vi "O2Scale.vi"() -> ()   [LabVIEW 2018]
uses:
  <vilib>/regexp/Match Regular Expression.xnode
panel:
  out "data out init 4":string="53 Ready for user\r\n"
  out "data out init 3":string="12 Access OK\r\n"
  in  "address 2":string="192.168.1.102"
  out "data out 4":string="00R614~       641.0~\r\n"
  in  "bytes to read 2":i32=100
  out "data out 3":string="00R615~       252.0~\r\n"
  out "East Scale\nWeight [lbs] 2":dbl(knob)=641.0 scale=0.0..800.0
  out "O2 East\nWeight [lbs] 2":dbl(knob)=252.0 scale=0.0..600.0
  out "O2 West\nWeight [lbs]":dbl(knob)=252.0 scale=0.0..600.0
  out "West Scale\nWeight [lbs]":dbl(knob)=641.0 scale=0.0..800.0
  in  "address":string="192.168.1.101"
  out "data out 2":string="00R131~       252.0~\r\n"
  in  "bytes to read":i32=100
  in  "stop":bool
  in  "milliseconds to wait":u32=1000
  out "data out 1":string="00R130~       641.0~\r\n"
  out "data out init 2":string="12 Access OK\r\n"
  out "data out init 1":string="53 Ready for user\r\n"
  # "53 Ready for user"
  # "12 Access OK"
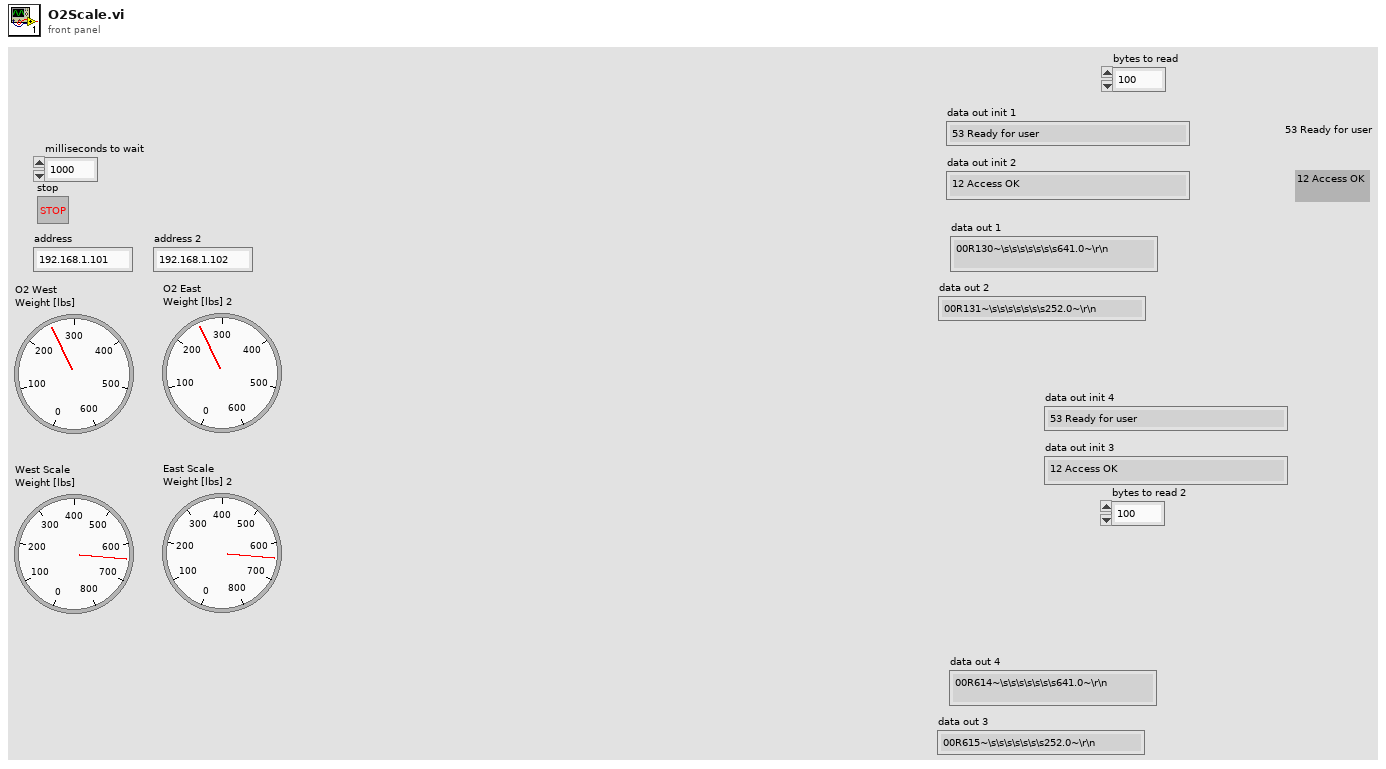
[diagram p1: front panel]
types:
  T1 = enum16{"open", "open or create", "create or replace", "create", "open (read-only)"}
  T2 = enum16{"Standard", "Buffered", "CRLF", "Immediate"}
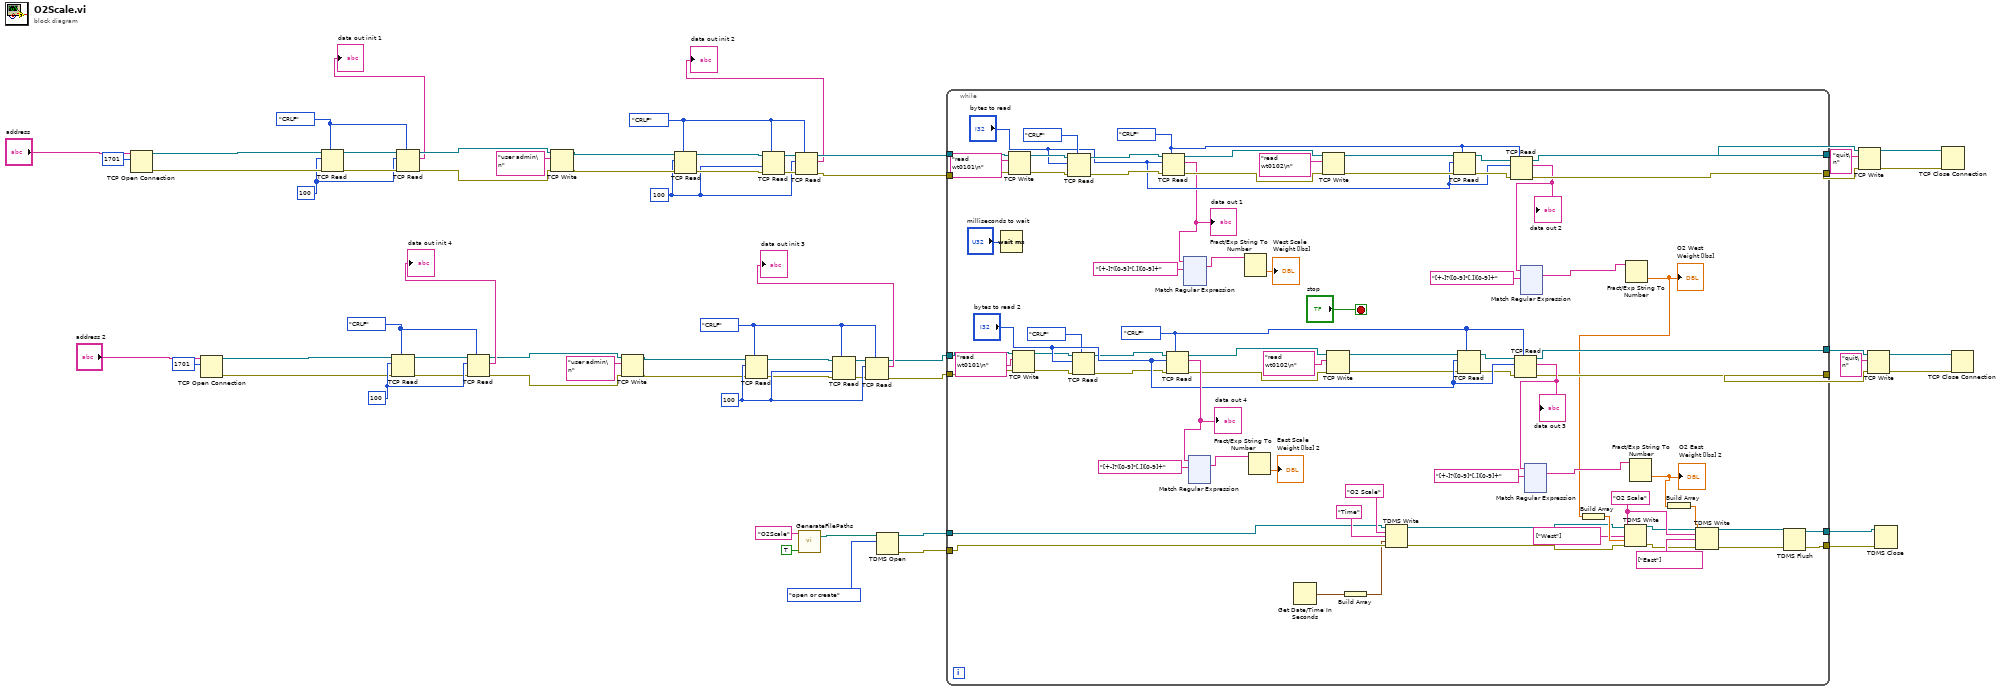
[diagram p0: block diagram]
diagram:
  w34 = 100 ("bytes to read")
  w35 = T2."CRLF" ("mode (standard)")
  w30 = 100 ("bytes to read")
  w25 = T2."CRLF" ("mode (standard)")
  w39 = 100 ("bytes to read")
  w38 = T2."CRLF" ("mode (standard)")
  w45 = 100 ("bytes to read")
  w50 = T2."CRLF" ("mode (standard)")
  n1 = TCP Open Connection(address="address", remote port or service name=u16 1701) -> (connection ID=w62:refnum<k5>, error out=w61:errorcluster)  [unwired: 3 in]
  n2 = TCP Open Connection(address="address 2", remote port or service name=u16 1701) -> (connection ID=w18:refnum<k5>, error out=w19:errorcluster)  [unwired: 3 in]
  n3 = TCP Read(connection ID=w62, bytes to read=w45, error in (no error)=w61, 7:w50) -> (connection ID out=w49:refnum<k5>, error out=w48:errorcluster)  [unwired: 1 in, 1 out]
  n4 = TCP Read(connection ID=w18, bytes to read=w30, error in (no error)=w19, 7:w25) -> (connection ID out=w26:refnum<k5>, error out=w27:errorcluster)  [unwired: 1 in, 1 out]
  n5 = TCP Read(connection ID=w49, bytes to read=w45, error in (no error)=w48, 7:w50) -> (connection ID out=w47:refnum<k5>, data out=→"data out init 1":string, error out=w46:errorcluster)  [unwired: 1 in]
  n6 = TCP Read(connection ID=w26, bytes to read=w30, error in (no error)=w27, 7:w25) -> (connection ID out=w28:refnum<k5>, data out=→"data out init 4":string, error out=w29:errorcluster)  [unwired: 1 in]
  n7 = TCP Write(connection ID=w47, data in="user admin\n", error in (no error)=w46) -> (connection ID out=w59:refnum<k5>, error out=w58:errorcluster)  [unwired: 1 in, 1 out]
  n8 = TCP Write(connection ID=w28, data in="user admin\n", error in (no error)=w29) -> (connection ID out=w21:refnum<k5>, error out=w22:errorcluster)  [unwired: 1 in, 1 out]
  n9 = TCP Read(connection ID=w59, bytes to read=w39, error in (no error)=w58, 7:w38) -> (connection ID out=w52:refnum<k5>, error out=w51:errorcluster)  [unwired: 1 in, 1 out]
  n10 = TCP Read(connection ID=w21, bytes to read=w34, error in (no error)=w22, 7:w35) -> (connection ID out=w23:refnum<k5>, error out=w24:errorcluster)  [unwired: 1 in, 1 out]
  n11 = TCP Read(connection ID=w52, error in (no error)=w51, 7:w38, 9:w39) -> (connection ID out=w42:refnum<k5>, error out=w43:errorcluster)  [unwired: 1 in, 1 out]
  n12 = TCP Read(connection ID=w42, bytes to read=w39, error in (no error)=w43, 7:w38) -> (connection ID out=w41:refnum<k5>, data out=→"data out init 2":string, error out=w40:errorcluster)  [unwired: 1 in]
  n13 = call "GenerateFilePaths.vi"("Logfile? (F)"=TRUE, "Device Name"="O2Scale") -> ("Path"=w6:path)  [unwired: 3 in]
  n14 = TCP Read(connection ID=w23, error in (no error)=w24, 7:w35, 9:w34) -> (connection ID out=w33:refnum<k5>, error out=w32:errorcluster)  [unwired: 1 in, 1 out]
  n15 = TCP Read(connection ID=w33, bytes to read=w34, error in (no error)=w32, 7:w35) -> (connection ID out=w15:refnum<k5>, data out=→"data out init 3":string, error out=w14:errorcluster)  [unwired: 1 in]
  n16 = TDMS Open(10:T1."open or create" ("operation (0:open)"), 11:w6) -> (0:w4:errorcluster, 3:w5:refnum<k34>)  [unwired: 5 in]
  n17 = while {
    tunnel: w41 -> [w139]
    tunnel: w40 -> [w138]
    tunnel: [w122] -> w53
    tunnel: [w121] -> w54
    tunnel: w15 -> [w89]
    tunnel: w14 -> [w88]
    tunnel: [w87] -> w10
    tunnel: [w86] -> w9
    tunnel: w5 -> [w65]
    tunnel: w4 -> [w71]
    tunnel: [w74] -> w3
    tunnel: [w73] -> w2
    stop <- "stop" stop-if-true
    w83 = "O2 Scale" ("group name in (Untitled)")
    w93 = T2."CRLF" ("mode (standard)")
    w120 = T2."CRLF" ("mode (standard)")
    n18 = Wait (ms)(milliseconds to wait="milliseconds to wait") -> ()  [unwired: 1 out]
    n19 = TCP Write(connection ID=w139, data in="read wt0101\n", error in (no error)=w138) -> (connection ID out=w137:refnum<k5>, error out=w136:errorcluster)  [unwired: 1 in, 1 out]
    n20 = TCP Write(connection ID=w89, data in="read wt0101\n", error in (no error)=w88) -> (connection ID out=w96:refnum<k5>, error out=w97:errorcluster)  [unwired: 1 in, 1 out]
    n21 = TCP Read(connection ID=w137, bytes to read="bytes to read", error in (no error)=w136, 7:T2."CRLF" ("mode (standard)")) -> (connection ID out=w128:refnum<k5>, error out=w127:errorcluster)  [unwired: 1 in, 1 out]
    n22 = TCP Read(connection ID=w96, bytes to read="bytes to read 2", error in (no error)=w97, 7:T2."CRLF" ("mode (standard)")) -> (connection ID out=w100:refnum<k5>, error out=w101:errorcluster)  [unwired: 1 in, 1 out]
    n23 = TCP Read(connection ID=w128, bytes to read="bytes to read", error in (no error)=w127, 7:w120) -> (connection ID out=w126:refnum<k5>, data out=w118:string, error out=w125:errorcluster)  [unwired: 1 in]
    "data out 1" <- w118
    n24 = TCP Read(connection ID=w100, bytes to read="bytes to read 2", error in (no error)=w101, 7:w93) -> (connection ID out=w102:refnum<k5>, data out=w107:string, error out=w103:errorcluster)  [unwired: 1 in]
    "data out 4" <- w107
    n25 = xnode "Match Regular Expression"("input string"=w118, "regular expression"="[+-]?([0-9]*[.])[0-9]+") -> ("whole match"=w114:string)  [unwired: 4 in, 4 out]
    n26 = xnode "Match Regular Expression"("input string"=w107, "regular expression"="[+-]?([0-9]*[.])[0-9]+") -> ("whole match"=w109:string)  [unwired: 4 in, 4 out]
    n27 = Fract/Exp String To Number(string=w114) -> (number=→"West Scale\nWeight [lbs]":dbl)  [unwired: 3 in, 1 out]
    n28 = Fract/Exp String To Number(string=w109) -> (number=→"East Scale\nWeight [lbs] 2":dbl)  [unwired: 3 in, 1 out]
    n29 = Get Date/Time In Seconds() -> (seconds since 1Jan1904=w70:timestamp)
    n30 = TCP Write(connection ID=w126, data in="read wt0102\n", error in (no error)=w125) -> (connection ID out=w130:refnum<k5>, error out=w131:errorcluster)  [unwired: 1 in, 1 out]
    n31 = TCP Write(connection ID=w102, data in="read wt0102\n", error in (no error)=w103) -> (connection ID out=w99:refnum<k5>, error out=w98:errorcluster)  [unwired: 1 in, 1 out]
    n32 = Build Array(w70) -> (w69:timestamp[])
    n33 = TDMS Write(0:w65, 5:"O2 Scale" ("group name in (Untitled)"), 7:"Time", 9:w69, 11:w71) -> (4:w66:refnum<k34>, 15:w72:errorcluster)  [unwired: 1 in, 2 out]
    n34 = TCP Read(connection ID=w130, bytes to read="bytes to read", error in (no error)=w131, 7:w120) -> (connection ID out=w124:refnum<k5>, error out=w123:errorcluster)  [unwired: 1 in, 1 out]
    n35 = TCP Read(connection ID=w99, bytes to read="bytes to read 2", error in (no error)=w98, 7:w93) -> (connection ID out=w104:refnum<k5>, error out=w105:errorcluster)  [unwired: 1 in, 1 out]
    n36 = TCP Read(connection ID=w124, bytes to read="bytes to read", error in (no error)=w123, 7:w120) -> (connection ID out=w122:refnum<k5>, data out=w115:string, error out=w121:errorcluster)  [unwired: 1 in]
    "data out 2" <- w115
    n37 = TCP Read(connection ID=w104, bytes to read="bytes to read 2", error in (no error)=w105, 7:w93) -> (connection ID out=w87:refnum<k5>, data out=w108:string, error out=w86:errorcluster)  [unwired: 1 in]
    "data out 3" <- w108
    n38 = xnode "Match Regular Expression"("input string"=w115, "regular expression"="[+-]?([0-9]*[.])[0-9]+") -> ("whole match"=w112:string)  [unwired: 4 in, 4 out]
    n39 = xnode "Match Regular Expression"("input string"=w108, "regular expression"="[+-]?([0-9]*[.])[0-9]+") -> ("whole match"=w111:string)  [unwired: 4 in, 4 out]
    n40 = Fract/Exp String To Number(string=w112) -> (number=w85:dbl)  [unwired: 3 in, 1 out]
    "O2 West\nWeight [lbs]" <- w85
    n41 = Build Array(w85) -> (w84:dbl[])
    n42 = TDMS Write(0:w66, 5:w83, 7:string[] ["West"] ("channel name(s) in (Untitled)"), 9:w84, 11:w72) -> (4:w78:refnum<k34>, 15:w76:errorcluster)  [unwired: 1 in, 2 out]
    n43 = Fract/Exp String To Number(string=w111) -> (number=w80:dbl)  [unwired: 3 in, 1 out]
    "O2 East\nWeight [lbs] 2" <- w80
    n44 = Build Array(w80) -> (w79:dbl[])
    n45 = TDMS Write(0:w78, 5:w83, 7:string[] ["East"] ("channel name(s) in (Untitled)"), 9:w79, 11:w76) -> (4:w77:refnum<k34>, 15:w75:errorcluster)  [unwired: 1 in, 2 out]
    n46 = TDMS Flush(4:w75, 7:w77) -> (0:w73:errorcluster, 3:w74:refnum<k34>)
  }
  n47 = TCP Write(connection ID=w53, data in="quit\n", error in (no error)=w54) -> (connection ID out=w56:refnum<k5>, error out=w55:errorcluster)  [unwired: 1 in, 1 out]
  n48 = TCP Write(connection ID=w10, data in="quit\n", error in (no error)=w9) -> (connection ID out=w12:refnum<k5>, error out=w13:errorcluster)  [unwired: 1 in, 1 out]
  n49 = TDMS Close(8:w2, 11:w3) -> ()  [unwired: 2 out]
  n50 = TCP Close Connection(connection ID=w56, error in (no error)=w55) -> ()  [unwired: 1 in, 2 out]
  n51 = TCP Close Connection(connection ID=w12, error in (no error)=w13) -> ()  [unwired: 1 in, 2 out]
